vi "Setpoint Type.vi"(8 "error in (no error)":errorcluster, 11 "Setpoint Function":T1) -> (0 "error out":errorcluster, 3 "Test Type":string)   [LabVIEW 2020]
uses:
  Controls/Serpoint.ctl
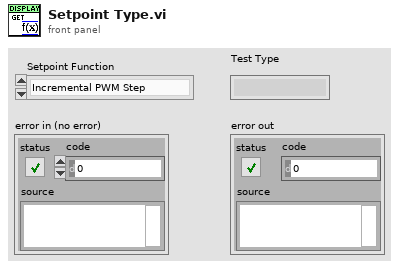
[diagram p1: front panel]
types:
  T1 = typedef "Serpoint.ctl" = enum16{"Incremental PWM Step", "PWM Step", "Ramp", "Sinusoidal", "Blood-Pressure"}
  T2 = cluster{"Setpoint Function":T1, "Test Type":string}[]
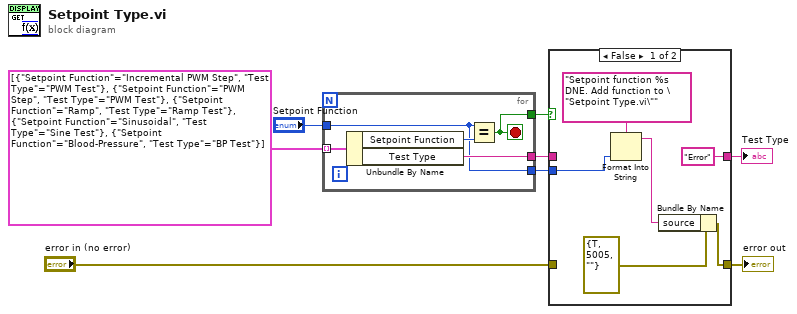
[diagram p0: block diagram]
diagram:
  n1 = for {
    tunnel: "Setpoint Function" -> [w9]
    tunnel: T2 [{"Setpoint Function"=enum."Incremental PWM Step", "Test Type"="PWM Test"}, {"Setpoint Function"=enum."PWM Step", "Test Type"="PWM Test"}, {"Setpoint Function"=enum."Ramp", "Test Type"="Ramp Test"}, {"Setpoint Function"=enum."Sinusoidal", "Test Type"="Sine Test"}, {"Setpoint Function"=enum."Blood-Pressure", "Test Type"="BP Test"}] ("NewVal") -> [w13] mode=indexing
    tunnel: [w11] -> w6
    tunnel: [w10] -> w4
    tunnel: [w9] -> w1
    stop <- w10 stop-if-true
    n2 = Unbundle By Name(w13) -> ("Setpoint Function"=w12:T1, "Test Type"=w11:string)
    n3 = Equal?(x=w9, y=w12) -> (x = y?=w10:bool)
  }
  n4 = case shown="False" w4 {
    tunnel: w6 -> [_ w21]
    tunnel: ["Error" ("Test Type") w21] -> w5
    tunnel: [w15 w20] -> w2
    tunnel: "error in (no error)" -> [_ w20]
    tunnel: w1 -> [w14 _]
    frame False {
      n5 = Format Into String(format string="Setpoint function %s DNE. Add function to \"Setpoint Type.vi\"", w14) -> (resulting string=w16:string)  [unwired: 2 in, 1 out]
      n6 = Bundle By Name(cluster=errorcluster {"status"=TRUE, "code"=5005, "source"=""} ("error constant"), "source"=w16) -> (w15:errorcluster)
    }
    frame True {
    }
  }
  "Test Type" <- w5
  "error out" <- w2
